vi "Towerlight.vi"(8 "error in":errorcluster, 11 "Notifier in":refnum<notifier>) -> (0 "error out":errorcluster, 3 "Notifier out":refnum<notifier>)   [LabVIEW 2017]
uses:
  <vilib>/DAQmx/write.llb/DAQmx Write (Digital 1D Bool NChan 1Samp 1Line).vi
  GV/Towerlight GV.vi
  <vilib>/DAQmx/miscellaneous.llb/DAQmx Fill In Error Info.vi
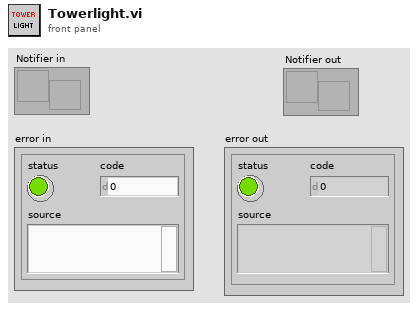
[diagram p1: front panel]
types:
  T1 = typedef "Towerlight.ctl" = enum16{"Idle", "Error", "Attention", "Running", "Maintenance", "Fail"}
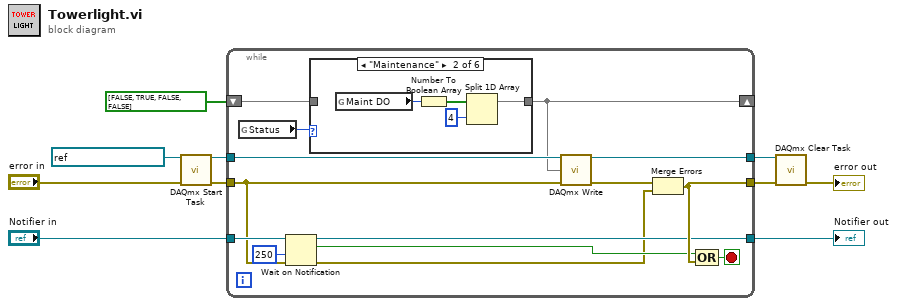
[diagram p0: block diagram]
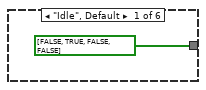
[diagram p2: hidden frame]
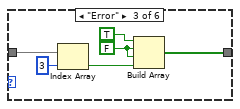
[diagram p3: hidden frame]
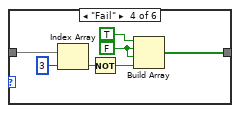
[diagram p4: hidden frame]
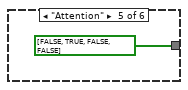
[diagram p5: hidden frame]
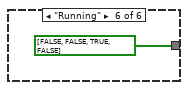
[diagram p6: hidden frame]
diagram:
  n1 = call <vilib>:"DAQmx Start Task.vi"("task/channels in"=refnum<k21> "1922_Towerlight", "error in"="error in") -> ("task out"=w3:refnum<k21>, "error out"=w1:errorcluster)  [unwired: 12 in]
  n2 = while {
    tunnel: w1 -> [w16]
    tunnel: w3 -> [w24]
    shift-right: [w12] -> _
    shift-left: bool[] [FALSE, TRUE, FALSE, FALSE] -> [w20]
    tunnel: [w22] -> w5
    tunnel: [w18] -> w6
    tunnel: "Notifier in" -> [w17]
    tunnel: [w13] -> w7
    stop <- w23 stop-if-true
    n3 = global read "Towerlight GV.vi" "Status"() -> (w21:T1)
    n4 = Wait on Notification(notifier=w17, timeout in ms (-1)=250, error in (no error)=w16) -> (notifier out=w13:refnum<notifier>, notification=w14:bool, error out=w11:errorcluster)  [unwired: 1 in, 1 out]
    n5 = case shown="\"Maintenance\"" w21 {
      tunnel: w20 -> [_ _ w35 w42 _ _]
      tunnel: [bool[] [FALSE, TRUE, FALSE, FALSE] w28 w32 w38 bool[] [FALSE, TRUE, FALSE, FALSE] bool[] [FALSE, FALSE, TRUE, FALSE]] -> w12
      frame "Idle", Default {
      }
      frame "Maintenance" {
        n6 = global read "Towerlight GV.vi" "Maint DO"() -> (w29:u32)
        n7 = Number To Boolean Array(number=w29) -> (Boolean array=w27:bool[])
        n8 = Split 1D Array(array=w27, index=4) -> (first subarray=w28:bool[])  [unwired: 1 out]
      }
      frame "Error" {
        w31 = FALSE ("element")
        n9 = Index Array(array=w35, index=3) -> (element=w30:bool)
        n10 = Build Array(TRUE, w31, w31, w30) -> (w32:bool[])
      }
      frame "Fail" {
        w37 = FALSE ("element")
        n11 = Index Array(array=w42, index=3) -> (element=w40:bool)
        n12 = Not(x=w40) -> (.not. x?=w36:bool)
        n13 = Build Array(TRUE, w37, w37, w36) -> (w38:bool[])
      }
      frame "Attention" {
      }
      frame "Running" {
      }
    }
    n14 = call-poly <vilib>:"DAQmx Write.vi"("task/channels in"=w24, "data"=w12, "error in"=w16) -> ("task out"=w22:refnum<k21>, "error out"=w19:errorcluster)  [unwired: 10 in, 1 out]
    n15 = Merge Errors(w19, w11) -> (w18:errorcluster)
    n16 = Compound Arithmetic op=OR(w14, w18) -> (w23:bool)
  }
  "Notifier out" <- w7
  n17 = call <vilib>:"DAQmx Clear Task.vi"("task in"=w5, "error in"=w6) -> ("error out"=→"error out":errorcluster)  [unwired: 13 in]
